vi "Check IP address.vi"(8 "error in (no error)":errorcluster, 11 "IP string":string) -> (0 "error out":errorcluster, 3 "Got all fields and data good?":bool)   [LabVIEW 2013]
panel:
  out "4th good?":bool
  out "3rd good?":bool
  out "2nd good?":bool
  out "1st good?":bool
  out "4th":string
  out "3rd":string
  out "2nd":string
  out "1st":string
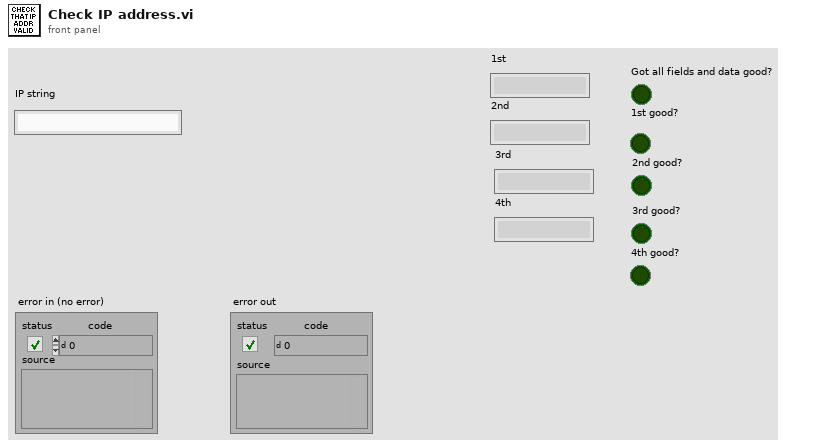
[diagram p1: front panel]
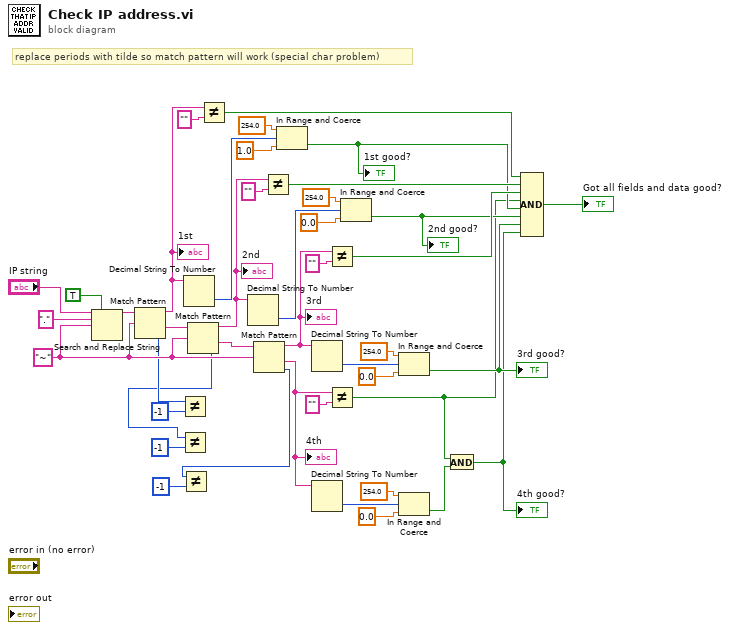
[diagram p0: block diagram]
diagram:
  w39 = "~" ("replace string (\"\")")
  # "replace periods with tilde so match pattern will work (special char problem)"
  n1 = Search and Replace String(replace all?=TRUE ("replace all? (F)"), input string="IP string", search string="." ("regular expression"), replace string=w39) -> (result string=w38:string)  [unwired: 4 in, 3 out]
  n2 = Match Pattern(string=w38, regular expression=w39) -> (before substring=w26:string, after substring=w43:string, offset past match=w9:i32)  [unwired: 1 in, 1 out]
  "1st" <- w26
  n3 = Not Equal?(x=w9, y=-1) -> ()  [unwired: 1 out]
  n4 = Decimal String To Number(string=w26) -> (number=w25:i32)  [unwired: 2 in, 1 out]
  n5 = Match Pattern(string=w43, regular expression=w39) -> (before substring=w15:string, after substring=w42:string, offset past match=w5:i32)  [unwired: 1 in, 1 out]
  "2nd" <- w15
  n6 = Not Equal?(x=w5, y=-1) -> ()  [unwired: 1 out]
  n7 = Not Equal?(x=w26, y="") -> (x != y?=w32:bool)
  n8 = Decimal String To Number(string=w15) -> (number=w24:i32)  [unwired: 2 in, 1 out]
  n9 = Match Pattern(string=w42, regular expression=w39) -> (before substring=w14:string, after substring=w13:string, offset past match=w4:i32)  [unwired: 1 in, 1 out]
  "3rd" <- w14
  "4th" <- w13
  n10 = Not Equal?(x=w4, y=-1) -> ()  [unwired: 1 out]
  n11 = Not Equal?(x=w15, y="") -> (x != y?=w31:bool)
  n12 = In Range and Coerce(upper limit=254.0, x=w25, lower limit=1.0) -> (In Range?=w12:bool)  [unwired: 1 out]
  "1st good?" <- w12
  n13 = Decimal String To Number(string=w14) -> (number=w19:i32)  [unwired: 2 in, 1 out]
  n14 = Decimal String To Number(string=w13) -> (number=w18:i32)  [unwired: 2 in, 1 out]
  n15 = Not Equal?(x=w14, y="") -> (x != y?=w30:bool)
  n16 = Not Equal?(x=w13, y="") -> (x != y?=w3:bool)
  n17 = In Range and Coerce(upper limit=254.0, x=w24, lower limit=0.0) -> (In Range?=w11:bool)  [unwired: 1 out]
  "2nd good?" <- w11
  n18 = In Range and Coerce(upper limit=254.0, x=w19, lower limit=0.0) -> (In Range?=w10:bool)  [unwired: 1 out]
  "3rd good?" <- w10
  n19 = In Range and Coerce(upper limit=254.0, x=w18, lower limit=0.0) -> (In Range?=w2:bool)  [unwired: 1 out]
  n20 = And(x=w3, y=w2) -> (x .and. y?=w1:bool)
  "4th good?" <- w1
  n21 = Compound Arithmetic op=AND(w32, w31, w30, w3, w12, w11, w10, w1) -> (→"Got all fields and data good?":bool)
